vi "VisualizePPS.vi"() -> ()   [LabVIEW 2018, in "Visualization.lvlib" / "VisualizeAcPwr.lvclass"]
doc: "This VI listens for any measurement data associated with the provided PluginName and displays it to the user for analysis. The display is only suitable for data coming from thePacific Power Supply Plugin."
uses:
  VisualizeAcPwr.lvclass
  VisualizeBase/VisualizeBase_class/Requests/VisUserEventType.ctl
  <vilib>/event_ctls.llb/usereventprio.ctl
  AcPwr/AcPwrShared/clMeasurmentData.ctl
  <extravilib>/ChannelInstances/Tag-bool/Read With Abort.vi
  <extravilib>/ChannelInstances/Tag-bool/Write With Abort.vi
  <extravilib>/ChannelInstances/Tag-bool/Instantiate.vi
  <extravilib>/ChannelInstances/Tag-bool/EndpointRead.vi
  <vilib>/Utility/error.llb/Error Cluster From Error Code.vi
  <extravilib>/ChannelInstances/Tag-bool/Endpoint.vi
  <vilib>/ErrorRing/Error Ring.xnode
  VisualizeBase/VisualizeBase_class/VisualizeBase.lvclass
  <userlib>/NIST/NISTErrorLib/NISTErrorLib.lvlib
  AcPwr/AcPwrShared/AcPwrShared.lvlib
  <extravilib>/ChannelInstances/Tag-bool.lvlib
panel:
  out "PPS":waveform(dbl)[](graph)=[{"t0"=timestamp(3657200531.6397257 s since 1904-01-01), "dt"=1.0, "Y"=[46.19]}, {"t0"=timestamp(3657200531.6397257 s since 1904-01-01), "dt"=1.0, "Y"=[2.0]}, {"t0"=timestamp(3657200531.6397257 s since 1904-01-01), "dt"=1.0, "Y"=[60.0]}]
  out "Incorrect DataType?":bool
  in  "PluginName":string="AcPwr.PPS0"
  in  "btnStop":bool
  in  "btnReset":bool
  in  "btnClear":bool
  out "ErrorArray":errorcluster[](array[cluster])
  in  "PlotYAxis":u32[](array[numeric])=[0, 1, 0, 0] max=1
  in  "QueueName":string="PPSVQ"
  # "0=Left Axis and 1=Right Axis"
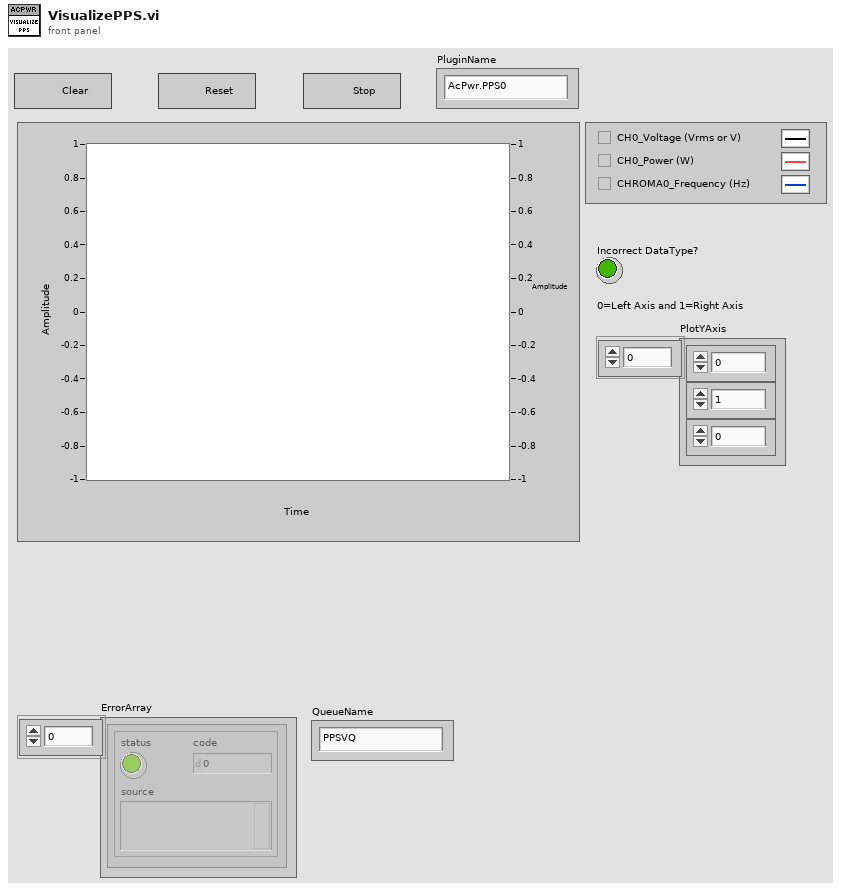
[diagram p1: front panel]
types:
  T1 = typedef "Visualization.lvlib/VisualizeBase.lvclass/VisRequestEvents.ctl" = cluster{"StopRequest":refnum<user-event>, "ResetRequest":refnum<user-event>, "FP Pop In or Out":refnum<user-event>}
  T2 = typedef "AcPwrShared.lvlib/AcPwrBroadcastEvents.ctl" = cluster{"DidInit":refnum<user-event>, "StatusUpdate":refnum<user-event>, "ErrorReport":refnum<user-event>, "DidStop":refnum<user-event>, "PathToINI":refnum<user-event>, "Measurements":refnum<user-event>, "LoadConfigFile":refnum<user-event>, "GetSettings":refnum<user-event>, "SetSettings":refnum<user-event>, "GetType&ID":refnum<user-event>, "GotSettings":refnum<user-event>}
  T3 = typedef "AcPwrShared.lvlib/clMeasurmentData.ctl" = cluster{"MeasName":string, "XML Data":string, "WaveformData":waveform(dbl)[]}
  T4 = typedef "Visualization.lvlib/VisualizeBase.lvclass/VisUserEventType.ctl" = cluster{"BusIndex":i8, "Data":variant}
  T5 = typedef "usereventprio.ctl" = enum32{"high priority", "normal priority"}
  T6 = typedef "Tag-bool.lvlib/))Channel.ctl" = refnum<queue>
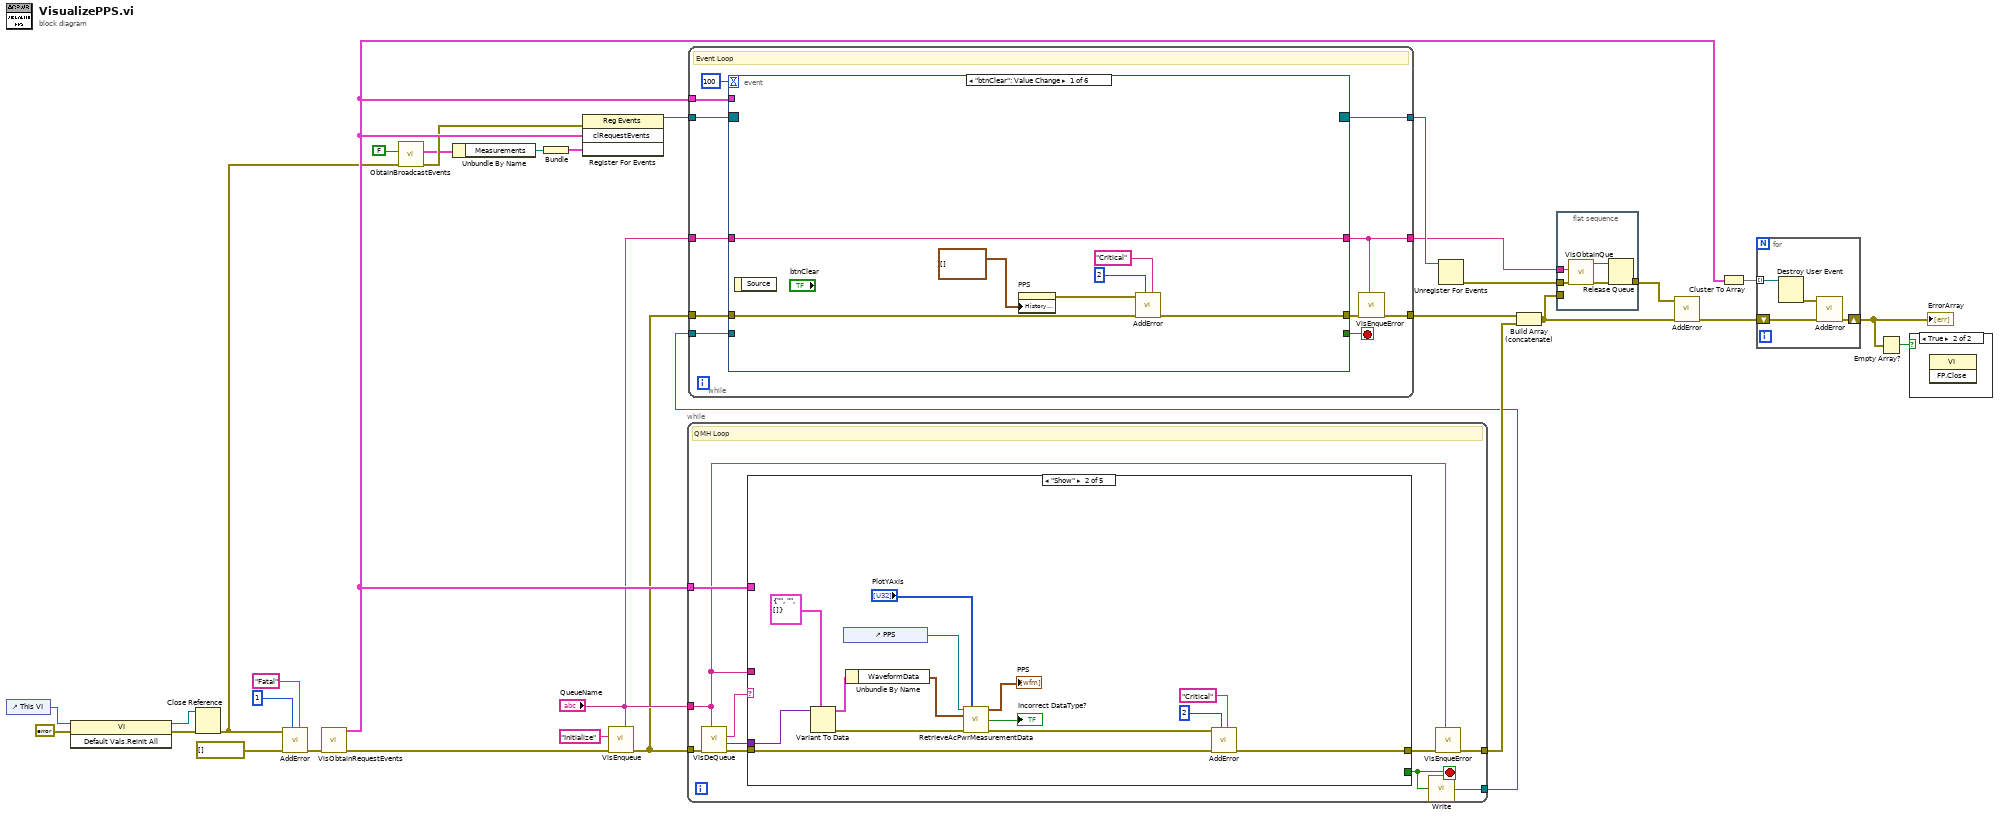
[diagram p0: block diagram]
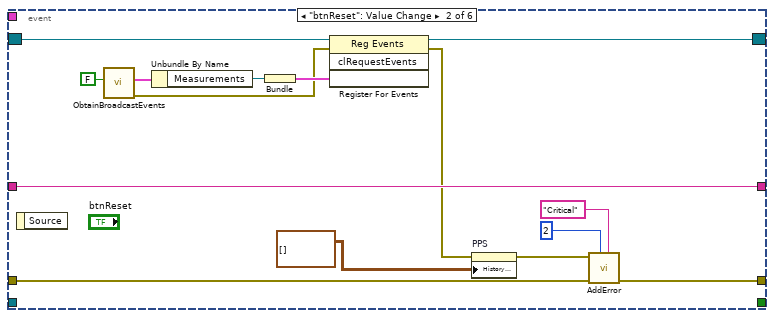
[diagram p2: hidden frame]
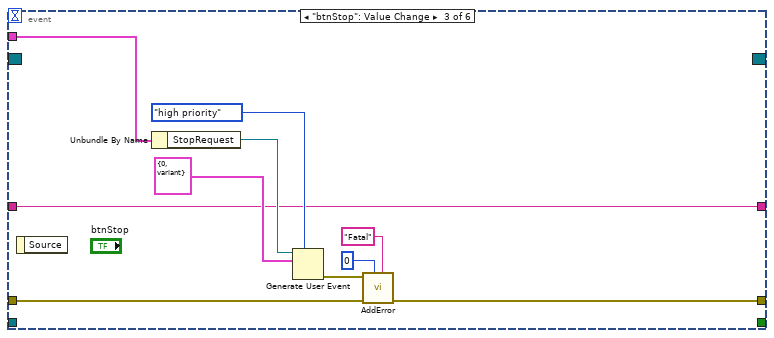
[diagram p3: hidden frame]
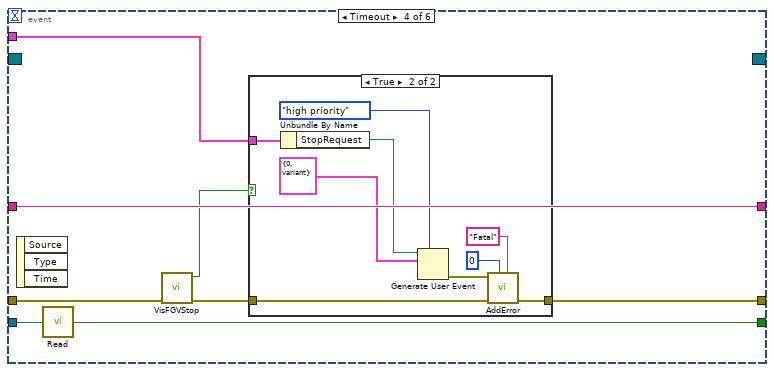
[diagram p4: hidden frame]
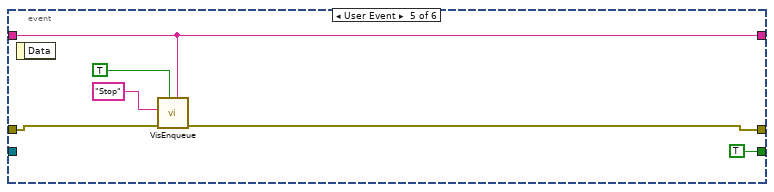
[diagram p6: hidden frame]
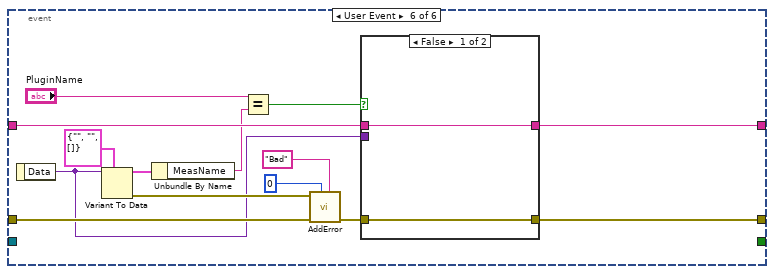
[diagram p7: hidden frame]
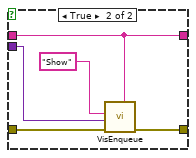
[diagram p8: hidden frame]
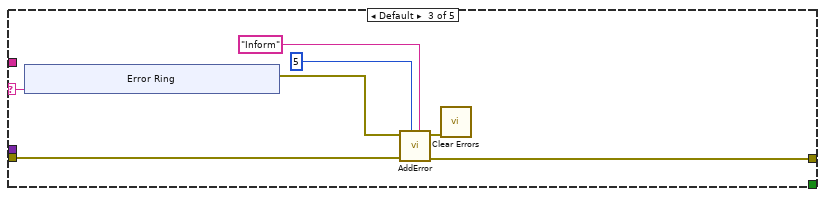
[diagram p10: hidden frame]
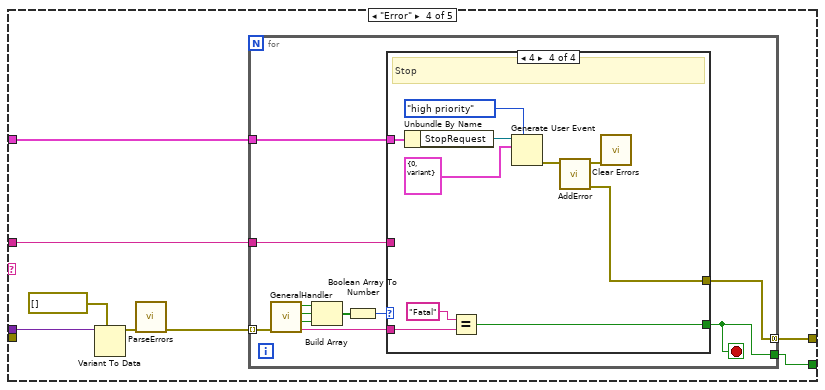
[diagram p11: hidden frame]
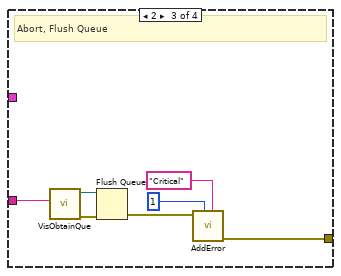
[diagram p14: hidden frame]
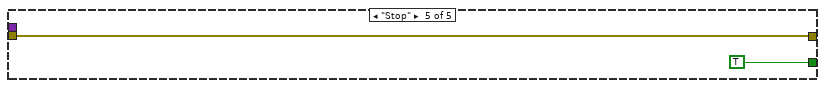
[diagram p15: hidden frame]
diagram:
  n1 = control-ref of="This VI"() -> (w17:refnum<vi>)
  n2 = invoke class="VI" method="Default Vals.Reinit All"(reference=w17, error in=errorcluster {"status"=FALSE, "code"=0, "source"=""} ("error in (no error)")) -> (reference out=w14:refnum<vi>, error out=w15:errorcluster)  [unwired: 1 in, 1 out]
  n3 = Close Reference(reference=w14, error in (no error)=w15) -> (error out=w5:errorcluster)
  n4 = call <userlib>:"AddError.vi"("Severity"="Fatal" ("String"), "Priority"=u8 1, "ErrorArray In"=errorcluster[] [] ("ErrorArray"), "error in (no error)"=w5) -> ("ErrorArray Out"=w30:errorcluster[])  [unwired: 6 in, 1 out]
  n5 = call "VisObtainRequestEvents.vi"("Error"=w30) -> ("Error"=w18:errorcluster[], "clRequestEvents"=w22:T1)  [unwired: 9 in]
  n6 = call "ObtainBroadcastEvents.vi"("error in (no error)"=w5, "CreateNew? (F)"=FALSE ("CreateNew (F)")) -> ("error out"=w3:errorcluster, "clAcPwrEvents"=w2:T2)  [unwired: 8 in]
  n7 = Unbundle By Name(w2) -> ("Measurements"=w20:refnum<user-event>)
  n8 = Bundle("Measurements"=w20) -> (w19:cluster{"Measurements":refnum<user-event>})  [unwired: 1 in]
  n9 = register-events(error in=w3, w22, w19) -> (reference out=w31:refnum<event-registration>)  [unwired: 1 in, 1 out]
  n10 = call "VisEnqueue.vi"("QueName"="QueueName", "Error"=w18, "Message"="Initialize") -> ("Error"=w8:errorcluster[])  [unwired: 8 in]
  n11 = while {
    tunnel: w8 -> [w42]
    tunnel: [w36] -> w26
    tunnel: "QueueName" -> [w34]
    tunnel: w22 -> [w35]
    tunnel: [w33] -> w1
    stop <- w37 stop-if-true
    # "QMH Loop"
    n12 = call "VisDeQueue.vi"("QueName"=w34, "Error"=w42) -> ("Error"=w39:errorcluster[], "Data"=w40:variant, "Message"=w41:string)  [unwired: 7 in]
    n13 = case shown="\"Show\"" w41 {
      selector: w41 -> [_ _ w64 _ _]
      tunnel: w40 -> [_ w56 _ w79 _]
      tunnel: w39 -> [w43 w53 w62 _ w108]
      tunnel: [w43 w57 w61 w75 w108] -> w38
      tunnel: [_ _ _ w74 TRUE] -> w37
      tunnel: w35 -> [_ _ _ w73 _]
      tunnel: w34 -> [_ _ _ w72 _]
      frame "Initialize" {
      }
      frame "Show" {
        n14 = Variant To Data(type=T3 {"MeasName"="", "XML Data"="", "WaveformData"=[]} ("MeasurmentDataCluster"), Variant=w56) -> (data=w46:T3, error out=w49:errorcluster)  [unwired: 1 in]
        n15 = control-ref of="PPS"() -> (w44:refnum<vi>)
        n16 = Unbundle By Name(w46) -> ("WaveformData"=w45:waveform(dbl)[])
        n17 = call "RetrieveAcPwrMeasurementData.vi"("WaveformChartReference"=w44, "PlotYScale"="PlotYAxis", "WaveformArrayIn"=w45, "error in (no error)"=w49) -> ("WaveformArrayOut"=→"PPS":waveform(dbl)[], "Incorrect DataType?"=→"Incorrect DataType?":bool, "error out"=w51:errorcluster)  [unwired: 7 in, 2 out]
        n18 = call <userlib>:"AddError.vi"("Severity"="Critical" ("String"), "Priority"=u8 2, "ErrorArray In"=w53, "error in (no error)"=w51) -> ("ErrorArray Out"=w57:errorcluster[])  [unwired: 6 in, 1 out]
      }
      frame Default {
        n19 = xnode "Error Ring"("parameter 0"=w64) -> ("error out"=w63:errorcluster)
        n20 = call <userlib>:"AddError.vi"("Severity"="Inform" ("String"), "Priority"=u8 5, "ErrorArray In"=w62, "error in (no error)"=w63) -> ("ErrorArray Out"=w61:errorcluster[], "error out"=w60:errorcluster)  [unwired: 6 in]
        n21 = call <vilib>:"Clear Errors.vi"("error in (no error)"=w60) -> ()  [unwired: 5 in, 2 out]
      }
      frame "Error" {
        n22 = Variant To Data(type=errorcluster[] [], Variant=w79) -> (data=w77:errorcluster[])  [unwired: 1 in, 1 out]
        n23 = call <userlib>:"ParseErrors.vi"("ErrorArray"=w77) -> ("ErrorArray"=w76:errorcluster[])  [unwired: 8 in, 2 out]
        n24 = for {
          tunnel: w76 -> [w90] mode=indexing
          tunnel: [w84] -> w75 mode=concatenating
          tunnel: [w82] -> w74
          tunnel: w73 -> [w81]
          tunnel: w72 -> [w80]
          stop <- w82 stop-if-true
          n25 = call <userlib>:"GeneralHandler.vi"("error in (no error)"=w90) -> ("Severity"=w83:string, "Stop"=w87:bool, "Abort"=w88:bool, "Continue"=w89:bool)  [unwired: 6 in, 1 out]
          n26 = Build Array(w89, w88, w87) -> (w86:bool[])
          n27 = Boolean Array To Number(Boolean array=w86) -> (number=w85:u32)
          n28 = case shown="4" w85 {
            tunnel: [_ _ w95 w106] -> w84
            tunnel: w83 -> [_ _ _ w101]
            tunnel: [_ _ _ w99] -> w82
            tunnel: w81 -> [_ _ _ w98]
            tunnel: w80 -> [_ _ w91 _]
            frame 0, Default {
              # "No Dialog"
            }
            frame 1 {
              # "Continue"
            }
            frame 2 {
              # "Abort, Flush Queue"
              n29 = call "VisObtainQue.vi"("QueName"=w91) -> ("error out"=w97:errorcluster, "queue out"=w96:refnum<queue>)  [unwired: 9 in]
              n30 = Flush Queue(queue=w96, error in (no error)=w97) -> (error out=w94:errorcluster)  [unwired: 2 out]
              n31 = call <userlib>:"AddError.vi"("Severity"="Critical" ("String"), "Priority"=u8 1, "error in (no error)"=w94) -> ("ErrorArray Out"=w95:errorcluster[])  [unwired: 7 in, 1 out]
            }
            frame 4 {
              # "Stop"
              n32 = Unbundle By Name(w98) -> ("StopRequest"=w107:refnum<user-event>)
              n33 = Equal?(x="Fatal", y=w101) -> (x = y?=w99:bool)
              n34 = Generate User Event(priority (normal)=usereventprio."high priority", user event=w107, event data cluster=T4 {"BusIndex"=0, "Data"=variant} ("event data")) -> (error out=w105:errorcluster)  [unwired: 1 in, 1 out]
              n35 = call <userlib>:"AddError.vi"("error in (no error)"=w105) -> ("ErrorArray Out"=w106:errorcluster[], "error out"=w102:errorcluster)  [unwired: 9 in]
              n36 = call <vilib>:"Clear Errors.vi"("error in (no error)"=w102) -> ()  [unwired: 5 in, 2 out]
            }
          }
        }
      }
      frame "Stop" {
      }
    }
    n37 = call <extravilib>:"Write.vi"("element"=w37) -> ("channel"=w33:T6)  [unwired: 1 out]
    n38 = call "VisEnqueError.vi"("QueName"=w34, "Error"=w38) -> ("Error"=w36:errorcluster[])  [unwired: 9 in]
  }
  n39 = while {
    tunnel: w31 -> [w120]
    tunnel: [w117] -> w27
    tunnel: [w116] -> w29
    tunnel: w22 -> [w115]
    tunnel: w8 -> [w114]
    tunnel: "QueueName" -> [w113]
    tunnel: [w112] -> w12
    tunnel: w1 -> [w110]
    stop <- w119 stop-if-true
    # "Event Loop"
    n40 = event shown="[0] \"btnClear\": Value Change" {
      selector: w120 -> [_ w142 _ _ _ _]
      dyn-events: [_ w141 _ _ _ _] -> w116
      timeout: 100 -> [_ _ _ _ _ _]
      tunnel: [_ _ _ w153 TRUE _] -> w119
      tunnel: [w123 w134 w150 w160 w175 w190] -> w118
      tunnel: w115 -> [_ _ w145 w159 _ _]
      tunnel: w114 -> [w124 w135 w143 w157 w172 w183]
      tunnel: w113 -> [w127 w136 w144 w158 w171 w189]
      tunnel: [w127 w136 w144 w158 w171 w184] -> w112
      tunnel: w110 -> [_ _ _ w154 _ _]
      event "btnClear": Value Change {
        n41 = event-data() -> ()  [unwired: 1 in, 1 out]
        n42 = property on="PPS" class="WFChart (strict)"("History Data"=waveform(dbl)[][] []) -> (error out=w122:errorcluster)  [unwired: 2 in, 1 out]
        n43 = call <userlib>:"AddError.vi"("Severity"="Critical" ("String"), "Priority"=u8 2, "ErrorArray In"=w124, "error in (no error)"=w122) -> ("ErrorArray Out"=w123:errorcluster[])  [unwired: 6 in, 1 out]
      }
      event "btnReset": Value Change {
        n44 = event-data() -> ()  [unwired: 1 in, 1 out]
        n45 = call "ObtainBroadcastEvents.vi"("CreateNew? (F)"=FALSE) -> ("error out"=w137:errorcluster, "clAcPwrEvents"=w138:T2)  [unwired: 9 in]
        n46 = Unbundle By Name(w138) -> ("Measurements"=w140:refnum<user-event>)
        n47 = Bundle("Measurements"=w140) -> (w139:cluster{"Measurements":refnum<user-event>})  [unwired: 1 in]
        n48 = register-events(reference=w142, error in=w137, w139) -> (reference out=w141:refnum<event-registration>, error out=w131:errorcluster)  [unwired: 1 in]
        n49 = property on="PPS" class="WFChart (strict)"(error in=w131, "History Data"=waveform(dbl)[][] []) -> (error out=w130:errorcluster)  [unwired: 1 in, 1 out]
        n50 = call <userlib>:"AddError.vi"("Severity"="Critical" ("String"), "Priority"=u8 2, "ErrorArray In"=w135, "error in (no error)"=w130) -> ("ErrorArray Out"=w134:errorcluster[])  [unwired: 6 in, 1 out]
      }
      event "btnStop": Value Change {
        n51 = event-data() -> ()  [unwired: 1 in, 1 out]
        n52 = Unbundle By Name(w145) -> ("StopRequest"=w151:refnum<user-event>)
        n53 = Generate User Event(priority (normal)=usereventprio."high priority", user event=w151, event data cluster=T4 {"BusIndex"=0, "Data"=variant} ("event data")) -> (error out=w152:errorcluster)  [unwired: 1 in, 1 out]
        n54 = call <userlib>:"AddError.vi"("Severity"="Fatal" ("String"), "Priority"=u8 0, "ErrorArray In"=w143, "error in (no error)"=w152) -> ("ErrorArray Out"=w150:errorcluster[])  [unwired: 6 in, 1 out]
      }
      event Timeout {
        n55 = event-data() -> ()  [unwired: 1 in, 3 out]
        n56 = call <extravilib>:"Read.vi"("channel"=w154) -> ("element"=w153:bool)  [unwired: 1 in, 1 out]
        n57 = call "VisFGVStop.vi"("Error In"=w157) -> ("Error Out"=w156:errorcluster[], "Value"=w155:bool)  [unwired: 9 in]
        n58 = case shown="True" w155 {
          tunnel: [w161 w168] -> w160
          tunnel: w159 -> [_ w163]
          tunnel: w156 -> [w161 w162]
          frame False {
          }
          frame True {
            n59 = Unbundle By Name(w163) -> ("StopRequest"=w169:refnum<user-event>)
            n60 = Generate User Event(priority (normal)=usereventprio."high priority", user event=w169, event data cluster=T4 {"BusIndex"=0, "Data"=variant} ("event data")) -> (error out=w170:errorcluster)  [unwired: 1 in, 1 out]
            n61 = call <userlib>:"AddError.vi"("Severity"="Fatal" ("String"), "Priority"=u8 0, "ErrorArray In"=w162, "error in (no error)"=w170) -> ("ErrorArray Out"=w168:errorcluster[])  [unwired: 6 in, 1 out]
          }
        }
      }
      event User Event {
        n62 = event-data() -> ()  [unwired: 1 in, 1 out]
        n63 = call "VisEnqueue.vi"("QueName"=w171, "Priority? (F)"=TRUE, "Error"=w172, "Message"="Stop") -> ("Error"=w175:errorcluster[])  [unwired: 7 in]
      }
      event User Event {
        n64 = event-data() -> ("Data"=w180:variant)  [unwired: 1 in]
        n65 = Variant To Data(type=T3 {"MeasName"="", "XML Data"="", "WaveformData"=[]} ("MeasurmentDataCluster"), Variant=w180) -> (data=w178:T3, error out=w186:errorcluster)  [unwired: 1 in]
        n66 = Unbundle By Name(w178) -> ("MeasName"=w177:string)
        n67 = Equal?(x="PluginName", y=w177) -> (x = y?=w182:bool)
        n68 = call <userlib>:"AddError.vi"("Severity"="Bad" ("String"), "Priority"=u8 0, "ErrorArray In"=w183, "error in (no error)"=w186) -> ("ErrorArray Out"=w185:errorcluster[])  [unwired: 6 in, 1 out]
        n69 = case shown="False" w182 {
          tunnel: [w192 w196] -> w190
          tunnel: w189 -> [w191 w194]
          tunnel: w185 -> [w192 w195]
          tunnel: [w191 w194] -> w184
          tunnel: w180 -> [_ w193]
          frame False {
          }
          frame True {
            n70 = call "VisEnqueue.vi"("QueName"=w194, "Error"=w195, "Data"=w193, "Message"="Show") -> ("Error"=w196:errorcluster[])  [unwired: 7 in]
          }
        }
      }
    }
    n71 = call "VisEnqueError.vi"("QueName"=w112, "Error"=w118) -> ("Error"=w117:errorcluster[])  [unwired: 9 in]
  }
  n72 = Unregister For Events(event registration refnum=w29) -> (error out=w25:errorcluster)  [unwired: 1 in]
  n73 = Build Array (concatenate)(w27, w26) -> (w6:errorcluster[])
  n74 = flat-sequence {
    tunnel: w25 -> [w202]
    tunnel: [w199] -> w24
    tunnel: w12 -> [w198]
    tunnel: w6 -> [_]
    frame #0 {
      n75 = call "VisObtainQue.vi"("error in (no error)"=w202, "QueName"=w198) -> ("error out"=w201:errorcluster, "queue out"=w200:refnum<queue>)  [unwired: 8 in]
      n76 = Release Queue(queue=w200, error in (no error)=w201) -> (error out=w199:errorcluster)  [unwired: 1 in, 2 out]
    }
  }
  n77 = call <userlib>:"AddError.vi"("ErrorArray In"=w6, "error in (no error)"=w24) -> ("ErrorArray Out"=w23:errorcluster[])  [unwired: 8 in, 1 out]
  n78 = Cluster To Array(cluster=w22) -> (array=w28:refnum<user-event>[])
  n79 = for {
    tunnel: w28 -> [w206] mode=indexing
    shift-right: [w205] -> w7
    shift-left: w23 -> [w204]
    n80 = Destroy User Event(user event=w206) -> (error out=w203:errorcluster)  [unwired: 1 in]
    n81 = call <userlib>:"AddError.vi"("ErrorArray In"=w204, "error in (no error)"=w203) -> ("ErrorArray Out"=w205:errorcluster[])  [unwired: 8 in, 1 out]
  }
  "ErrorArray" <- w7
  n82 = Empty Array?(array=w7) -> (empty?=w21:bool)
  n83 = case shown="True" w21 {
    frame False {
    }
    frame True {
      n84 = invoke class="VI" method="FP.Close"() -> ()  [unwired: 3 in, 3 out]
    }
  }
